vi "Detrend Tach Signal.vi"(7 "extension":T1(ring)=enum."symmetric ext.", 8 "synthesis filters":cluster{"lowpass":dbl[], "highpass":dbl[]}={"lowpass"=[-0.1294095225512602, 0.22414386804201353, 0.8365163037378076, 0.48296291314453393], "highpass"=[-0.4829629131445343, 0.8365163037378082, -0.22414386804201325, -0.12940952255126054]} {"highpass" format="%.2e"; "lowpass" format="%.2e"}, 9 "analysis filters":cluster{"lowpass":dbl[], "highpass":dbl[]}={"lowpass"=[0.4829629131445343, 0.8365163037378082, 0.22414386804201325, -0.12940952255126054], "highpass"=[-0.1294095225512602, -0.22414386804201353, 0.8365163037378076, -0.48296291314453393]} {"highpass" format="%.2e"; "lowpass" format="%.2e"}, 10 "detrend level (0.0)":dbl=0.2 min=0.0 max=1.0 step=0.01 format="%.2f", 11 "x[n]":dbl[](array[numeric]) format="%.2f") -> (0 "error out":errorcluster, 1 "trend":dbl[](array[numeric]) format="%.2f", 3 "detrend":dbl[](array[numeric]) format="%.2f")   [LabVIEW 2017, in "SoundVib_TachProcess.lvlib"]
doc: "Performs wavelet-transform based detrending."
uses:
  <vilib>/addons/Sound and Vibration/Order Analysis/Tach Process/SoundVib_TachProcess.lvlib
  <resource>/sndvib.dll
panel:
  # "Detrend Tach Signal"
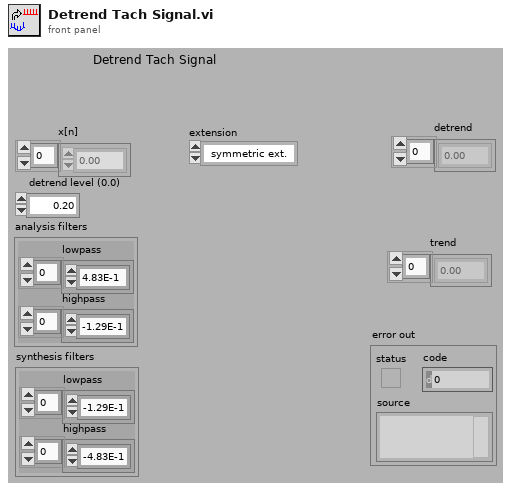
[diagram p1: front panel]
types:
  T1 = enum16{"zero padding", "symmetric ext.", "periodic ext.", "1st derivative", "2nd derivative"}
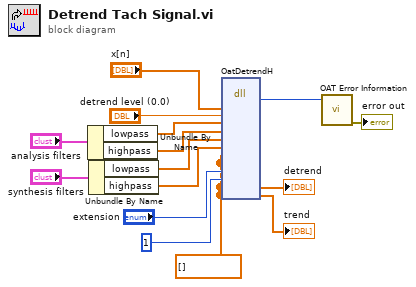
[diagram p0: block diagram]
diagram:
  w4 = dbl[] [] ("Array")
  n1 = Unbundle By Name("analysis filters") -> ("lowpass"=w12:dbl[], "highpass"=w11:dbl[])
  n2 = Unbundle By Name("synthesis filters") -> ("lowpass"=w9:dbl[], "highpass"=w8:dbl[])
  n3 = dll-call lib="C:/Program Files (x86)/National Instruments/LabVIEW 2017/resource/sndvib.*" fn="OatDetrendH"("xH"="x[n]", "level"="detrend level (0.0)", "a_lowpassH"=w12, "a_highpassH"=w11, "s_lowpassH"=w9, "s_highpassH"=w8, "initialCondition"=w4, "finalCondition"=w4, "extension"="extension", "shift"=1, "detrendH"=w4, "trendH"=w4) -> ("return type"=w2:i32, "detrendH"=→"detrend":dbl[], "trendH"=→"trend":dbl[])  [unwired: 13 in, 2 out]
  n4 = call <vilib>:"OAT Error Information.vi"("error code"=w2) -> ("error out"=→"error out":errorcluster)  [unwired: 6 in]
